vi "Set Test Executive Version.vi"(8 "error in (no error)":errorcluster, 11 "Test Executive Ref":refnum<data-value>) -> (0 "error out":errorcluster, 3 "Test Executive Ref out":refnum<data-value>)   [LabVIEW 2019, in "Test Executive.lvlib" / "TestExecutive Ref.lvclass"]
uses:
  <vilib>/gpm_packages/@cs/test-executive/Source/Test Executive/TestExecutive Ref/TestExecutive Ref.lvclass
  <vilib>/gpm_packages/@cs/test-executive/Source/Test Executive/ITestExecutive/ITest Executive.lvclass
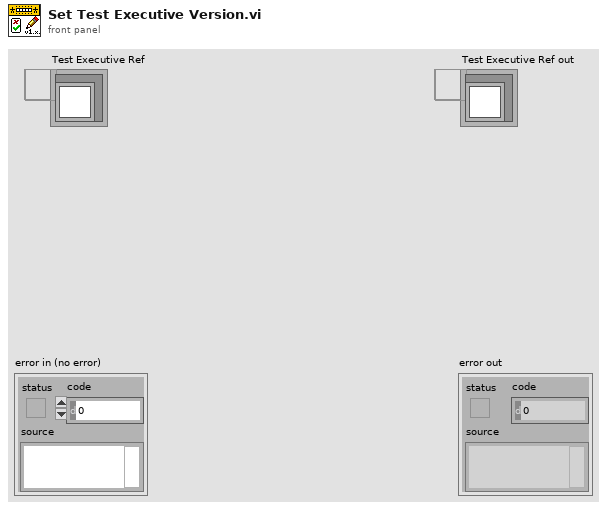
[diagram p1: front panel]
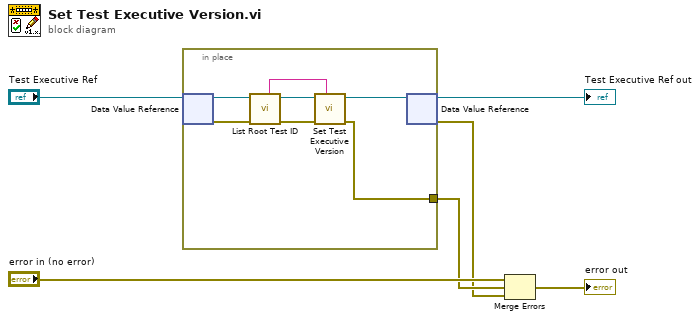
[diagram p0: block diagram]
diagram:
  n1 = in-place {
    in-place-border: [w12] -> w3
    n2 = in-place-dvr #1("Test Executive Ref") -> (w11:refnum<class "ITest Executive.lvclass">, w9:errorcluster)
    n3 = call-dynamic "List Root Test ID.vi"("error in (no error)"=w9, "ITest Executive in"=w11) -> ("error out"=w8:errorcluster, "ITest Executive out"=w10:refnum<class "ITest Executive.lvclass">, "Root ID"=w7:string)  [unwired: 5 in, 2 out]
    n4 = call-dynamic "Set Test Executive Version.vi"("Unique ID"=w7, "error in (no error)"=w8, "ITest Executive in"=w10) -> ("error out"=w12:errorcluster, "ITest Executive out"=w13:refnum<class "ITest Executive.lvclass">)  [unwired: 7 in]
    n5 = in-place-dvr #1(w13) -> (→"Test Executive Ref out":refnum<data-value>, w2:errorcluster)
  }
  n6 = Merge Errors("error in (no error)", w3, w2) -> (→"error out":errorcluster)
